vi "Rx.vi"() -> ()   [LabVIEW 2017]
uses:
  <vilib>/addons/Modulation/Analog/support/mod_Set Error Source.vi
  <vilib>/addons/Modulation/Digital/General/MT Generate PSK System Parameters(M).vi
  <vilib>/addons/Modulation/Digital/General/MT Generate PSK Synchronization Parameters (bit array).vi
  <vilib>/addons/Modulation/Digital/Support/Common/Validators/mod_Generate Filter Coefficients Validate.vi
  <vilib>/addons/Modulation/Digital/General/subVIs/mod_Generate Filter Coefficients.vi
  <vilib>/addons/Modulation/Digital/General/MT Generate Bits (Fibonacci, PN Order).vi
  <instrlib>/niUSRP/niUSRP Fetch Rx Data (CDB Cluster).vi
  <vilib>/addons/Modulation/Digital/Channel Coding/MT Convolutional Decoder (Viterbi Hard Decision, Rate).vi
  <vilib>/addons/Modulation/Digital/Demodulation/MT Calculate BER After Trigger (Fibonacci PN Sequence).vi
  <vilib>/addons/Modulation/niDMT.lvlib
panel:
  out "accumulated BER":dbl format="%.4f"
  out "BER":dbl format="%.4f"
  out "Received Signal":cluster{"t0":dbl, "dt":dbl, "Y":dbl[]}(graph)
  out "Constellation Graph":T1(graph) caption="Constellation Graph 2"
  in  "active antenna":string
  in  "stop":bool
  in  "gain":dbl format="%#_6f"
  in  "carrier frequency":dbl=100000.0 format="%#_6p"
  in  "IQ rate":dbl=100000.0 format="%#_6p"
  in  "device names":refnum<k15>
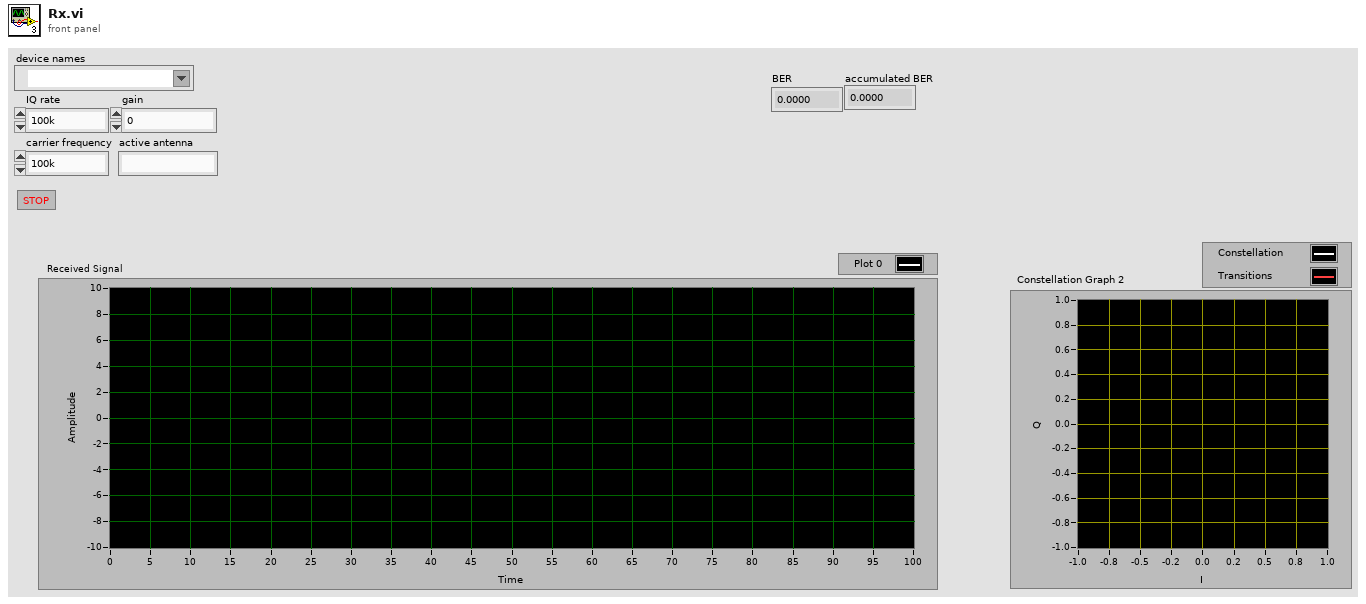
[diagram p1: front panel]
types:
  T1 = cluster{"Decimated Array":dbl[], "Decimated Array":dbl[]}[]
  T2 = enum16{"none", "Raised Cosine", "Root Raised Cos", "Gaussian"}
  T3 = enum16{"FSK", "PSK", "QAM", "MSK", "PAM", "ASK", "CPM"}
  T4 = cluster{"samples per symbol (16)":i32, "symbol map":cdb[], "differential PSK":enum16{"disable", "enable"}, "PSK type":u16}
  T5 = cluster{"expected sync location (symbols)":i32, "sync sequence":cdb[], "sync location uncertainty (symbols)":i32, "sync indent (symbols)":i32}
  T6 = cluster{"constellation":dbl[], "oversampled data":dbl[]}[]
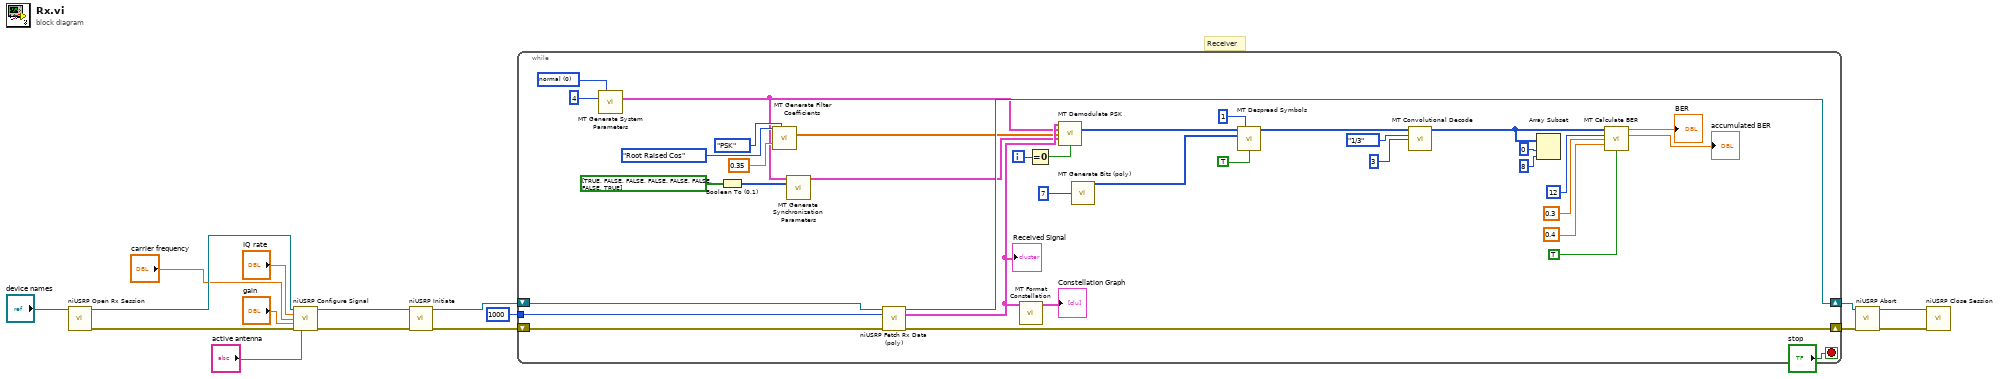
[diagram p0: block diagram]
diagram:
  # "Receiver"
  n1 = call <instrlib>:"niUSRP Open Rx Session.vi"("device names"="device names") -> ("session handle out"=w16:refnum<k15>, "error out"=w9:errorcluster)  [unwired: 13 in]
  n2 = call <instrlib>:"niUSRP Configure Signal.vi"("session handle"=w16, "IQ rate"="IQ rate", "carrier frequency"="carrier frequency", "gain"="gain", "error in (no error)"=w9, "active antenna"="active antenna") -> ("session handle out"=w15:refnum<k15>, "error out"=w10:errorcluster)  [unwired: 5 in, 3 out]
  n3 = call <instrlib>:"niUSRP Initiate.vi"("session handle"=w15, "error in (no error)"=w10) -> ("session handle out"=w4:refnum<k15>, "error out"=w3:errorcluster)  [unwired: 12 in]
  n4 = while {
    shift-right: [w52] -> w14
    shift-left: w4 -> [w53]
    shift-right: [w51] -> w11
    shift-left: w3 -> [w50]
    tunnel: i64 1000 ("number of samples") -> [w48]
    i -> [w24]
    stop <- "stop" stop-if-true
    w32 = u16 0 items=["normal", "shifted", "offset"] ("PSK type")
    n5 = call-poly <vilib>:"MT Generate System Parameters.vi"("PSK type"=w32, "M-PSK (4)"=4) -> ("PSK system parameters"=w17:T4)  [unwired: 11 in, 2 out]
    n6 = Boolean To (0,1)(Boolean=bool[] [TRUE, FALSE, FALSE, FALSE, FALSE, FALSE, FALSE, TRUE]) -> (0, 1=w33:i16[])
    n7 = call <vilib>:"MT Generate Filter Coefficients.vi"("pulse shaping filter (none)"=T2."Root Raised Cos", "modulation type"=T3."PSK", "filter parameter"=0.35) -> ("matched filter coefficients"=w19:dbl[])  [unwired: 10 in, 2 out]
    n8 = call-poly <vilib>:"MT Generate Synchronization Parameters.vi"("PSK system parameters"=w17, "sync bits"=w33) -> ("PSK synchronization parameters"=w18:T5)  [unwired: 12 in, 1 out]
    n9 = call-poly <instrlib>:"niUSRP Fetch Rx Data (poly).vi"("session handle"=w53, "number of samples"=w48, "error in (no error)"=w50) -> ("session handle out"=w52:refnum<k15>, "data"=w20:cluster{"t0":dbl, "dt":dbl, "Y":cdb[]}, "error out"=w51:errorcluster)  [unwired: 9 in, 1 out]
    "Received Signal" <- w20
    n10 = call <vilib>:"MT Format Constellation.vi"("waveform"=w20) -> ("constellation graph"=→"Constellation Graph":T6)  [unwired: 13 in, 1 out]
    n11 = Equal To 0?(x=w24) -> (x = 0?=w25:bool)
    n12 = call <vilib>:"MT Demodulate PSK.vi"("input complex waveform"=w20, "PSK system parameters"=w17, "matched filter coefficients"=w19, "synchronization parameters"=w18, "reset? (T)"=w25) -> ("output bit stream"=w46:i8[])  [unwired: 6 in, 4 out]
    n13 = call-poly <vilib>:"MT Generate Bits (poly).vi"("PN sequence order"=7) -> ("output bit stream"=w45:i8[])  [unwired: 12 in, 2 out]
    n14 = call <vilib>:"MT Despread Symbols.vi"("input chip stream"=w46, "sync search depth (bits)"=1, "spreading code"=w45, "reset? (T)"=TRUE) -> ("output bit stream"=w23:i8[])  [unwired: 8 in, 3 out]
    n15 = call-poly <vilib>:"MT Convolutional Decode.vi"("input bit stream"=w23, "rate (k/n)"=enum16{"1/2", "1/3", "1/4", "2/3", "3/4"}."1/3", "constraint length (K)"=3) -> ("output bit stream"=w47:i8[])  [unwired: 10 in, 2 out]
    n16 = Array Subset(array=w47, index=0, length=8) -> ()  [unwired: 1 out]
    n17 = call-poly <vilib>:"MT Calculate BER.vi"("input bit stream"=w47, "PN sequence order (9)"=12, "BER trigger threshold (0.1)"=0.3, "confidence (0.95)"=0.4, "reset? (T)"=TRUE) -> ("BER"=→"BER":dbl, "accumulated BER"=→"accumulated BER":dbl)  [unwired: 6 in, 3 out]
  }
  n18 = call <instrlib>:"niUSRP Abort.vi"("session handle"=w14, "error in (no error)"=w11) -> ("session handle out"=w13:refnum<k15>, "error out"=w12:errorcluster)  [unwired: 12 in]
  n19 = call <instrlib>:"niUSRP Close Session.vi"("session handle"=w13, "error in (no error)"=w12) -> ()  [unwired: 13 in, 1 out]
